vi "update file header for datapoint count.vi"(7 "Queues":T1, 11 "fileIO":T2) -> ()   [LabVIEW 2018]
uses:
  ICL-LabVIEW_General/data channels/data channels.lvlib
  supporting VIs/polymorphic VIs/enqueue for user interface.vi
  RT/Type Defs/channelScalingTypes.ctl
  RT/Type Defs/scalingMethods.ctl
  type defs/channelControl.ctl
  type defs/file IO data.ctl
  Chris VIs/data channels/parent class/Data Channel.lvclass
  type defs/Queues.ctl
panel:
  out "lastFile written":string
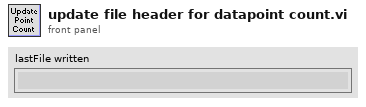
[diagram p1: front panel]
types:
  T1 = typedef "Queues.ctl" = cluster{"messageHandler":refnum<queue>, "comms":refnum<queue>, "dataStream":refnum<queue>, "dataProcessor":refnum<queue>, "fileIO":refnum<queue>, "userInterface":refnum<queue>, "errors":refnum<queue>, "customCompressor":refnum<queue>}
  T2 = typedef "file IO data.ctl" = cluster{"params":cluster{"startFolder":path, "channelConfigPath":path}, "vars":cluster{"channelConfig ":T3[], "writing":cluster{"streaming":bool, "fixedLength":bool, "pointCount":u32, "timeZero":dbl, "pointsWritten":u32, "dataRate":u16}, "channelCount":u16, "fileTarget":cluster{"Save folder":path, "Target filename":string, "file ref":refnum<file>, "pulsatorSpeed":string, "motorSpeed":string, "valvePosition":string, "torqueFilter":bool, "pulsatorRunning":bool, "motorRunning":bool}, "channels":refnum<class "Data Channel.lvclass">[]}}
  T3 = typedef "channelControl.ctl" = cluster{"index":u16, "active":bool, "channelType":T4, "module":u16, "terminal":u16, "channelName":string, "scalingMethod":T5, "scalingParameters":dbl[], "scaledUnits":string, "tempOffset":dbl}
  T4 = typedef "channelScalingTypes.ctl" = enum16{"calculation", "measurement", "scanivalve", "output", "digital"}
  T5 = typedef "scalingMethods.ctl" = enum16{"none", "linear", "thermocouple", "polynomial", "encoder", "RTD"}
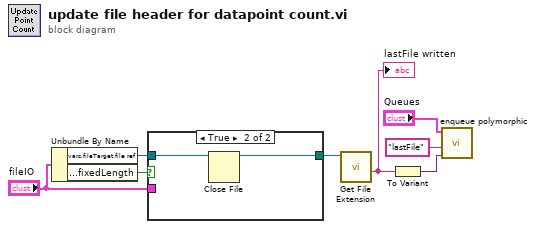
[diagram p0: block diagram]
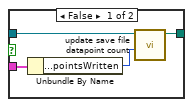
[diagram p2: hidden frame]
diagram:
  n1 = Unbundle By Name("fileIO") -> ("vars.fileTarget.file ref"=w8:refnum<file>, "vars.writing.fixedLength"=w7:bool)
  n2 = case shown="True" w7 {
    tunnel: w8 -> [w11 w14]
    tunnel: "fileIO" -> [w12 _]
    tunnel: [w9 w13] -> w4
    frame False {
      n3 = Unbundle By Name(w12) -> ("vars.writing.pointsWritten"=w10:u32)
      n4 = call "update save file datapoint count.vi"("pointsWritten"=w10, "fileRef"=w11) -> ("created file"=w9:path)  [unwired: 8 in, 1 out]
    }
    frame True {
      n5 = Close File(refnum=w14) -> (path=w13:path)  [unwired: 1 in, 1 out]
    }
  }
  n6 = call <vilib>:"Get File Extension.vi"("file"=w4) -> ("filename without extension"=w3:string)  [unwired: 6 in, 4 out]
  "lastFile written" <- w3
  n7 = To Variant(anything=w3) -> (Variant=w2:variant)
  n8 = call-poly "enqueue polymorphic.vi"("data"=w2, "message"="lastFile", "Queues"="Queues") -> ()  [unwired: 8 in, 1 out]
